vi "main.vi"() -> ()   [LabVIEW 2015]
uses:
  Stany_enum.ctl
  <vilib>/DAQmx/configure/timing.llb/DAQmx Timing (Use Waveform).vi
  <vilib>/DAQmx/create/channels.llb/DAQmx Create Channel (AO-Voltage-Basic).vi
  <vilib>/DAQmx/read.llb/DAQmx Read (Analog 1D DBL 1Chan NSamp).vi
  <resource>/objmgr/daqmx.rc
panel:
  in  "Sterowanie\naplikacją":cluster{"Start pomiaru":bool, "Stop":bool}
  out "Ostatni błąd":errorcluster
  in  "Ustawienia\npomiaru":T1={"Kanal pomiaru"="", "Czestotliwosc pomiaru"=1000.0, "Liczba probek na kanal pomiarowy"=1000} {"Czestotliwosc pomiaru" format="%0.2f"}
  in  "Ustawienia\ngeneratora":T2={"Kanal generatora"="", "Ksztalt sygnalu"=enum."Sine Wave", "RegenMode"=10097} {"RegenMode" items=["Allow Regeneration"=10097, "Do Not Allow Regeneration"=10158]}
  out "Generowany sygnal":waveform(dbl)(graph)
  out "Pomiar":dbl[](graph)
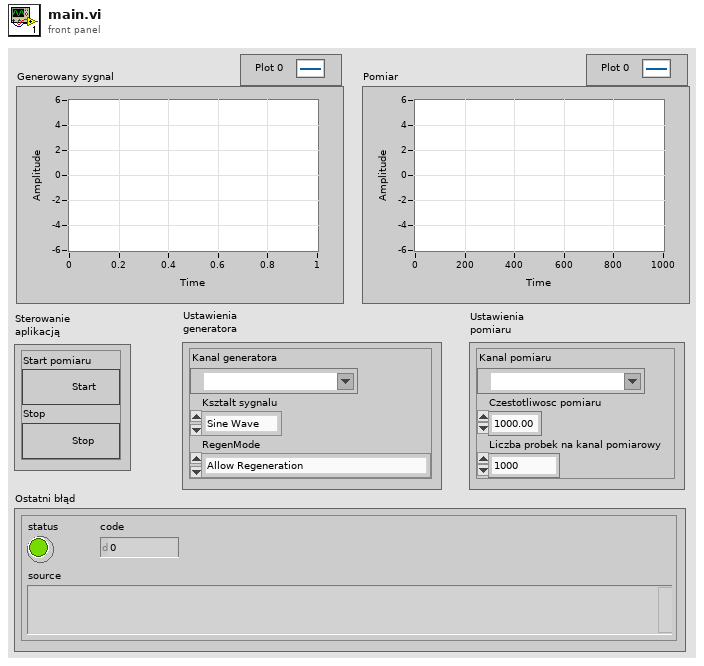
[diagram p1: front panel]
types:
  T1 = cluster{"Kanal pomiaru":tag, "Czestotliwosc pomiaru":dbl, "Liczba probek na kanal pomiarowy":i32}
  T2 = cluster{"Kanal generatora":tag, "Ksztalt sygnalu":enum16{"Sine Wave", "Triangle Wave", "Square Wave", "Sawtooth Wave"}, "RegenMode":i32}
  T3 = typedef "Stany_enum.ctl" = enum16{"Sprawdz czy STOP", "Czekaj na START", "Init", "Pracuj", "STOP", "Blad"}
  T4 = cluster{"RegenMode":refnum<vi>, "Ksztalt sygnalu":refnum<vi>, "Liczba probek na kanal pomiarowy":refnum<vi>, "Czestotliwosc pomiaru":refnum<vi>, "Kanal pomiaru":refnum<vi>, "Kanal generatora":refnum<vi>}
  T5 = enum8{"Enabled", "Disabled", "Disabled and Grayed Out"}
  T6 = enum16{"Sine Wave", "Triangle Wave", "Square Wave", "Sawtooth Wave"}
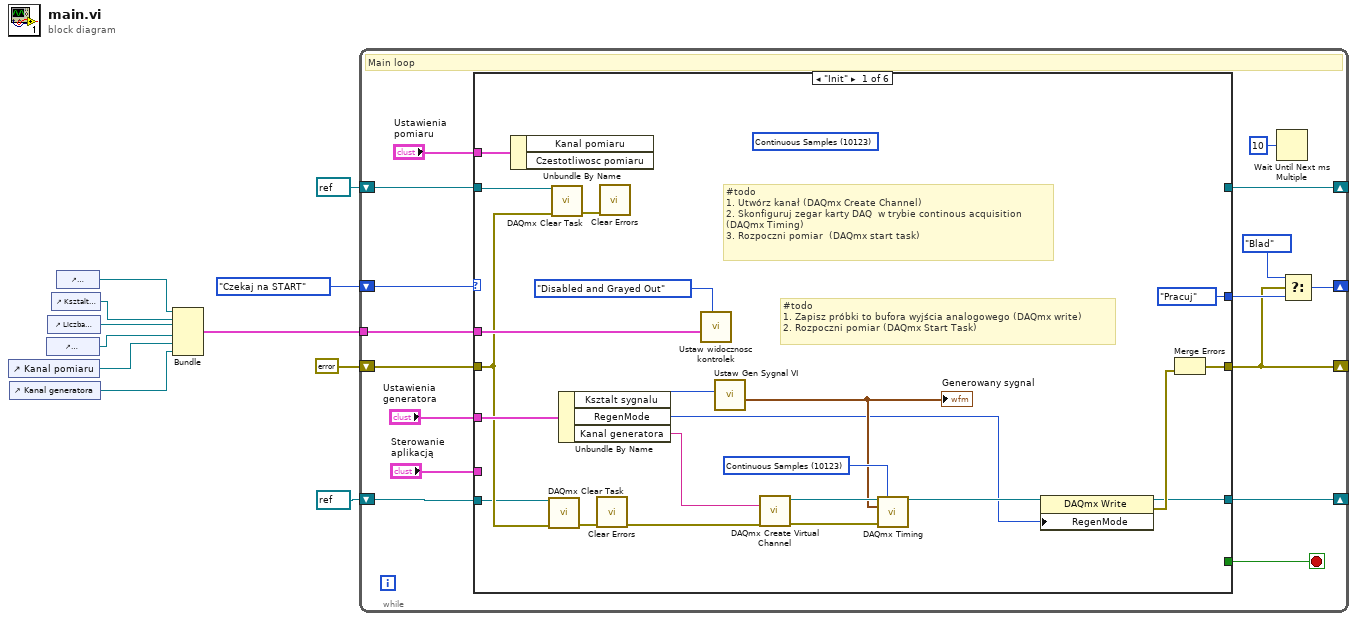
[diagram p0: block diagram]
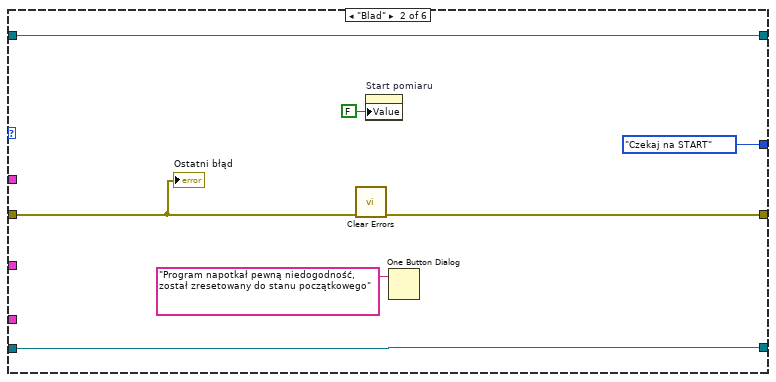
[diagram p2: hidden frame]
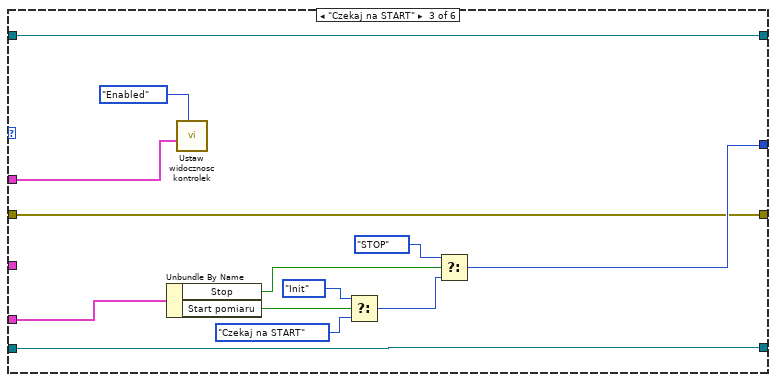
[diagram p3: hidden frame]
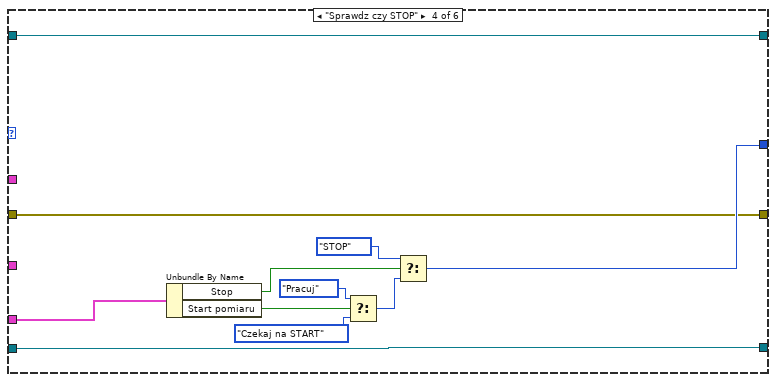
[diagram p4: hidden frame]
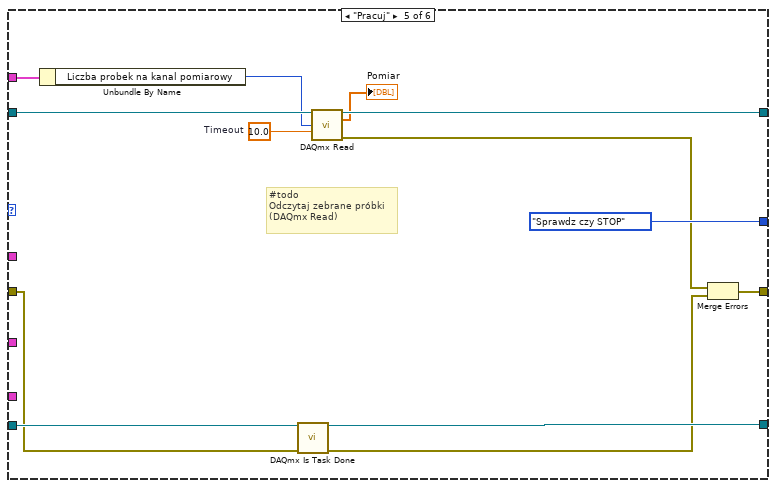
[diagram p5: hidden frame]
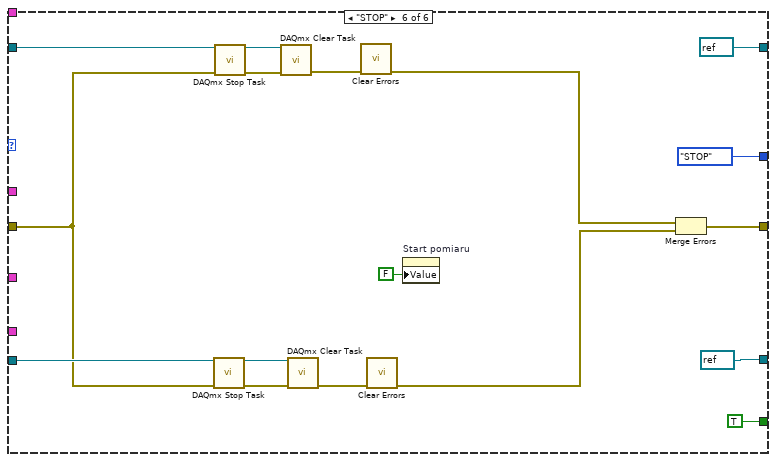
[diagram p6: hidden frame]
diagram:
  n1 = control-ref of="Kanal pomiaru"() -> (w3:refnum<vi>)
  n2 = control-ref of="Kanal generatora"() -> (w2:refnum<vi>)
  n3 = control-ref of="Czestotliwosc pomiaru"() -> (w4:refnum<vi>)
  n4 = control-ref of="Liczba probek na kanal pomiarowy"() -> (w5:refnum<vi>)
  n5 = control-ref of="Ksztalt sygnalu"() -> (w6:refnum<vi>)
  n6 = control-ref of="RegenMode"() -> (w7:refnum<vi>)
  n7 = Bundle("RegenMode"=w7, "Ksztalt sygnalu"=w6, "Liczba probek na kanal pomiarowy"=w5, "Czestotliwosc pomiaru"=w4, "Kanal pomiaru"=w3, "Kanal generatora"=w2) -> (w1:T4)  [unwired: 1 in]
  n8 = while {
    shift-right: [w26] -> _
    shift-left: refnum<k21> refnum ("task out") -> [w24]
    shift-right: [w25] -> _
    shift-left: refnum<k21> refnum ("task out") -> [w23]
    shift-right: [w17] -> _
    shift-left: Stany_enum."Czekaj na START" -> [w27]
    shift-right: [w18] -> _
    shift-left: errorcluster {"status"=FALSE, "code"=0, "source"=""} ("error out") -> [w20]
    tunnel: w1 -> [w12]
    stop <- w22 stop-if-true
    # "Main loop"
    n9 = case shown="\"Init\"" w27 {
      tunnel: [_ w55 w64 w71 w92 refnum<k21> refnum ("task out")] -> w26
      tunnel: [w28 w56 w65 w76 w90 refnum<k21> refnum ("task out")] -> w25
      tunnel: w24 -> [w32 w55 w64 w71 w93 w104]
      tunnel: w23 -> [w30 w56 w65 w76 w91 w101]
      tunnel: [Stany_enum."Pracuj" Stany_enum."Czekaj na START" w60 w72 Stany_enum."Sprawdz czy STOP" Stany_enum."STOP"] -> w19
      tunnel: [_ _ _ _ _ TRUE] -> w22
      tunnel: "Sterowanie\naplikacją" -> [_ _ w69 w80 _ _]
      tunnel: [w42 w54 w59 w70 w85 w96] -> w18
      tunnel: w20 -> [w31 w50 w59 w70 w86 w97]
      tunnel: "Ustawienia\ngeneratora" -> [w40 _ _ _ _ _]
      tunnel: "Ustawienia\npomiaru" -> [w39 _ _ _ w82 _]
      tunnel: w12 -> [w33 _ w58 _ _ _]
      frame "Init" {
        w48 = 10123 items=["Finite Samples"=10178, "Continuous Samples"=10123, "Hardware Timed Single Point"=12522] ("sample mode")
        (unwired) 10123 items=["Finite Samples"=10178, "Continuous Samples"=10123, "Hardware Timed Single Point"=12522] ("sample mode")
        # "#todo\n1. Zapisz próbki to bufora wyjścia analogowego (DAQmx write)\n2. Rozpoczni pomiar (DAQmx Start Task)"
        # "#todo\n1. Utwórz kanał (DAQmx Create Channel)\n2. Skonfiguruj zegar karty DAQ  w trybie continous acquisition\n(DAQmx Timing)\n3. Rozpoczni pomiar  (DAQmx start task)"
        n10 = Unbundle By Name(w39) -> ()  [unwired: 2 out]
        n11 = call <vilib>:"DAQmx Clear Task.vi"("task in"=w30, "error in"=w31) -> ("error out"=w44:errorcluster)  [unwired: 13 in]
        n12 = call <vilib>:"DAQmx Clear Task.vi"("task in"=w32, "error in"=w31) -> ("error out"=w45:errorcluster)  [unwired: 13 in]
        n13 = Unbundle By Name(w40) -> ("Ksztalt sygnalu"=w36:T6, "RegenMode"=w35:i32, "Kanal generatora"=w38:tag)
        n14 = call <vilib>:"Clear Errors.vi"("error in (no error)"=w44) -> ("error out"=w43:errorcluster)  [unwired: 5 in, 1 out]
        n15 = call <vilib>:"Clear Errors.vi"("error in (no error)"=w45) -> ()  [unwired: 5 in, 2 out]
        n16 = call "Ustaw widocznosc kontrolek.vi"("Disabled/Enabled"=T5."Disabled and Grayed Out" ("Disabled"), "Klaster referencji"=w33) -> ()  [unwired: 10 in]
        n17 = call "Ustaw Gen Sygnal VI.vi"("Ksztalt sygnalu"=w36) -> ("generowany sygnal"=w41:waveform(dbl))  [unwired: 10 in]
        "Generowany sygnal" <- w41
        n18 = call-poly <vilib>:"DAQmx Create Virtual Channel.vi"("physical channels"=w38, "error in"=w43) -> ("task out"=w47:refnum<k21>, "error out"=w49:errorcluster)  [unwired: 12 in]
        n19 = call-poly <vilib>:"DAQmx Timing.vi"("task/channels in"=w47, "sample mode"=w48, "waveform"=w41, "error in"=w49) -> ("task out"=w37:refnum<k21>)  [unwired: 10 in, 1 out]
        n20 = property class="DAQmx Write"(reference=w37, "RegenMode"=w35) -> (reference out=w28:refnum<k21>, error out=w29:errorcluster)  [unwired: 1 in]
        n21 = Merge Errors(w29) -> (w42:errorcluster)  [unwired: 1 in]
      }
      frame "Blad" {
        n22 = call <vilib>:"Clear Errors.vi"("error in (no error)"=w50) -> ("error out"=w54:errorcluster)  [unwired: 5 in, 1 out]
        n23 = property on="Start pomiaru" class="Bool (strict)"("Value"=FALSE) -> ()  [unwired: 2 in, 2 out]
        n24 = One Button Dialog(message="Program napotkał pewną niedogodność, został zresetowany do stanu początkowego") -> ()  [unwired: 1 in, 1 out]
        "Ostatni błąd" <- w50
      }
      frame "Czekaj na START" {
        n25 = Unbundle By Name(w69) -> ("Stop"=w63:bool, "Start pomiaru"=w68:bool)
        n26 = call "Ustaw widocznosc kontrolek.vi"("Disabled/Enabled"=T5."Enabled", "Klaster referencji"=w58) -> ()  [unwired: 10 in]
        n27 = Select(t=Stany_enum."Init", s=w68, f=Stany_enum."Czekaj na START") -> (s? t:f=w62:T3)
        n28 = Select(t=Stany_enum."STOP", s=w63, f=w62) -> (s? t:f=w60:T3)
      }
      frame "Sprawdz czy STOP" {
        n29 = Unbundle By Name(w80) -> ("Stop"=w75:bool, "Start pomiaru"=w79:bool)
        n30 = Select(t=Stany_enum."Pracuj", s=w79, f=Stany_enum."Czekaj na START") -> (s? t:f=w73:T3)
        n31 = Select(t=Stany_enum."STOP", s=w75, f=w73) -> (s? t:f=w72:T3)
      }
      frame "Pracuj" {
        w89 = 10.0  # Timeout
        # "#todo\nOdczytaj zebrane próbki\n(DAQmx Read)"
        n32 = Unbundle By Name(w82) -> ("Liczba probek na kanal pomiarowy"=w81:i32)
        n33 = call <vilib>:"DAQmx Is Task Done.vi"("task/channels in"=w91, "error in"=w86) -> ("task out"=w90:refnum<k21>, "error out"=w83:errorcluster)  [unwired: 11 in, 1 out]
        n34 = call-poly <vilib>:"DAQmx Read.vi"("task/channels in"=w93, "number of samples per channel"=w81, "timeout"=w89) -> ("task out"=w92:refnum<k21>, "data"=→"Pomiar":dbl[], "error out"=w84:errorcluster)  [unwired: 10 in]
        n35 = Merge Errors(w84, w83) -> (w85:errorcluster)
      }
      frame "STOP" {
        n36 = call <vilib>:"DAQmx Stop Task.vi"("task/channels in"=w101, "error in"=w97) -> ("task out"=w102:refnum<k21>, "error out"=w103:errorcluster)  [unwired: 12 in]
        n37 = call <vilib>:"DAQmx Stop Task.vi"("task/channels in"=w104, "error in"=w97) -> ("task out"=w106:refnum<k21>, "error out"=w105:errorcluster)  [unwired: 12 in]
        n38 = call <vilib>:"DAQmx Clear Task.vi"("task in"=w106, "error in"=w105) -> ("error out"=w99:errorcluster)  [unwired: 13 in]
        n39 = call <vilib>:"DAQmx Clear Task.vi"("task in"=w102, "error in"=w103) -> ("error out"=w98:errorcluster)  [unwired: 13 in]
        n40 = call <vilib>:"Clear Errors.vi"("error in (no error)"=w99) -> ("error out"=w95:errorcluster)  [unwired: 5 in, 1 out]
        n41 = call <vilib>:"Clear Errors.vi"("error in (no error)"=w98) -> ("error out"=w94:errorcluster)  [unwired: 5 in, 1 out]
        n42 = property on="Start pomiaru" class="Bool (strict)"("Value"=FALSE ("Start pomiaru")) -> ()  [unwired: 2 in, 2 out]
        n43 = Merge Errors(w95, w94) -> (w96:errorcluster)
      }
    }
    n44 = Wait Until Next ms Multiple(millisecond multiple=u32 10) -> ()  [unwired: 1 out]
    n45 = Select(t=Stany_enum."Blad", s=w18, f=w19) -> (s? t:f=w17:T3)
  }
